vi "temperatura con wfgraps.vi"() -> ()   [LabVIEW 2020]
panel:
  out "Waveform Chart":dynamicdata(graph)
  in  "stop":bool
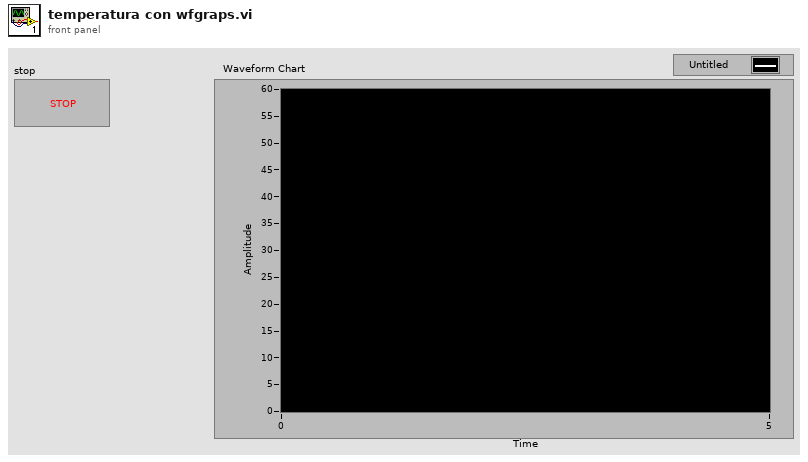
[diagram p1: front panel]
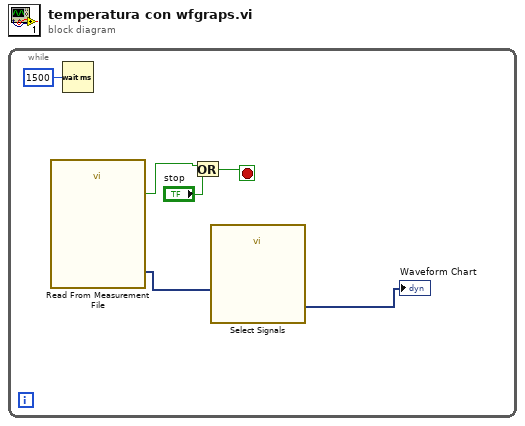
[diagram p0: block diagram]
diagram:
  n1 = while {
    stop <- w5 stop-if-true
    n2 = call "Read From Measurement File"() -> ("Signals"=w3:dynamicdata, "EOF?"=w2:bool)  [unwired: 6 in, 4 out]
    n3 = Wait (ms)(milliseconds to wait=u32 1500) -> ()  [unwired: 1 out]
    n4 = Or(x=w2, y="stop") -> (x .or. y?=w5:bool)
    n5 = call "Select Signals"("Signals"=w3) -> ("Signal Out"=→"Waveform Chart":dynamicdata)  [unwired: 9 in, 1 out]
  }
